vi "Get Listbox Text.vi"(8 "error in (no error)":errorcluster, 10 "bitfile path":path, 11 "Node Ptr":T1 format="%.0x") -> (0 "error out":errorcluster, 2 "Control Info":string[][](array[string]), 3 "Node Ptr out":T1 format="%.0x")   [LabVIEW 2013, in "PWM System Explorer.lvlib"]
uses:
  PWM System Explorer.lvlib
  <vilib>/NI Veristand/Custom Device API/Custom Device Item Ref.ctl
  Shared/Constants.vi
  <vilib>/regexp/Match Regular Expression.xnode
  Shared/PWM Shared.lvlib
  <vilib>/NI Veristand/Custom Device API/Custom Device API.lvlib
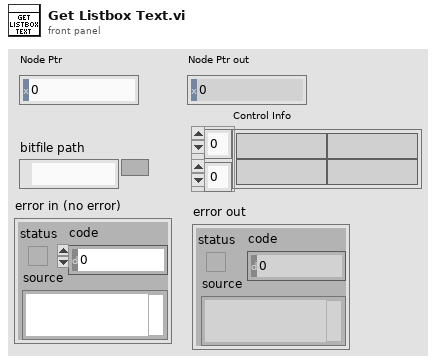
[diagram p1: front panel]
types:
  T1 = typedef "Custom Device API.lvlib/Custom Device Item Ref.ctl" = u64
  T2 = typedef "nirviReadCallControlInfo.ctl" = cluster{"names":string[], "indicator":bool[], "type descriptor":variant[], "size/rep":u32[], "top level type descriptor":variant[], "level":i32[], "class":string[], "address":i32[], "item orders":cluster{"order":u32[]}[], "name hierarchies":cluster{"name":string[]}[], "access may timeout":bool[], "from register node":bool[]}
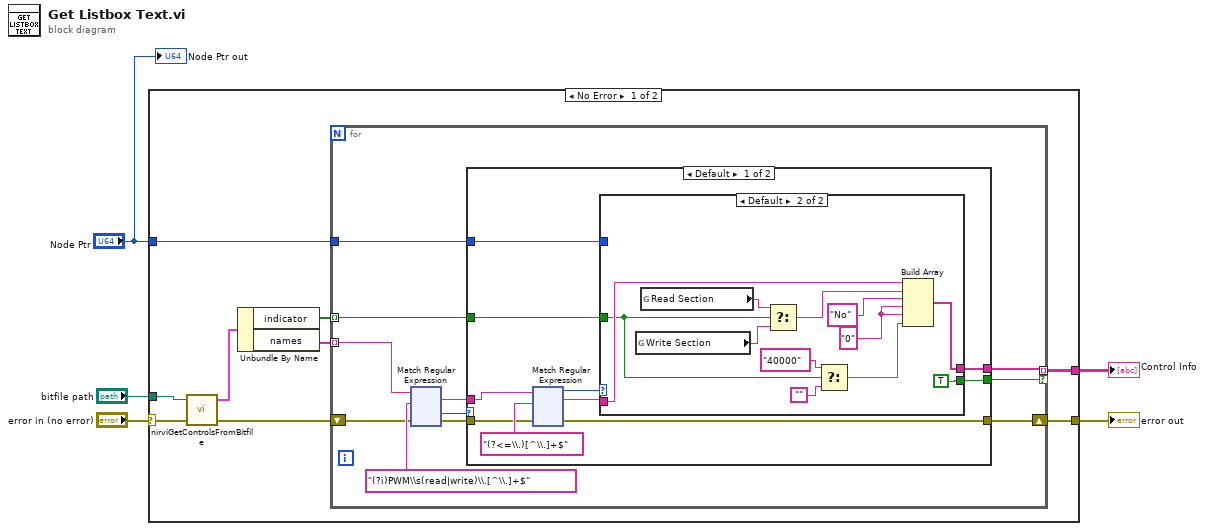
[diagram p0: block diagram]
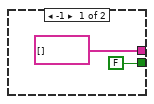
[diagram p2: hidden frame]
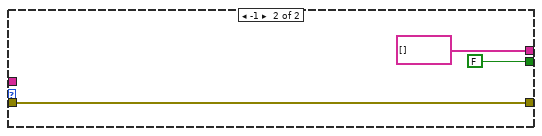
[diagram p3: hidden frame]
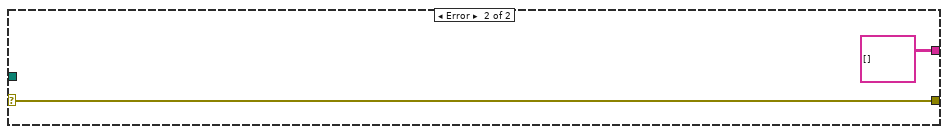
[diagram p4: hidden frame]
diagram:
  n1 = case shown="No Error" "error in (no error)" {
    selector: "error in (no error)" -> [w10 w282]
    tunnel: [w14 string[][] []] -> w5
    tunnel: "bitfile path" -> [w8 _]
    tunnel: [w11 w282] -> w2
    tunnel: "Node Ptr" -> [w6 _]
    frame No Error {
      n2 = call <vilib>:"nirviGetControlsFromBitfile.vi"("error in (no error)"=w10, "bitfile path"=w8) -> ("error out"=w9:errorcluster, "controls"=w12:T2)  [unwired: 2 in]
      n3 = Unbundle By Name(w12) -> ("indicator"=w13:bool[], "names"=w7:string[])
      n4 = for {
        tunnel: w7 -> [w25] mode=indexing
        tunnel: w13 -> [w21] mode=indexing
        tunnel: [w24] -> w14 mode=indexing if=w23
        shift-right: [w22] -> w11
        shift-left: w9 -> [w15]
        tunnel: w6 -> [w20]
        n5 = xnode "Match Regular Expression"("input string"=w25, "regular expression"="(?i)PWM\\s(read|write)\\.[^\\.]+$", "error in"=w15) -> ("whole match"=w17:string, "offset past match"=w19:i32, "error out"=w16:errorcluster)  [unwired: 3 in, 2 out]
        n6 = case shown="Default" w19 {
          tunnel: w21 -> [w35 _]
          tunnel: w17 -> [w30 _]
          tunnel: [w34 string[] []] -> w24
          tunnel: [w33 FALSE] -> w23
          tunnel: w20 -> [w28 _]
          tunnel: w16 -> [w27 w165]
          tunnel: [w26 w165] -> w22
          frame Default {
            n7 = xnode "Match Regular Expression"("input string"=w30, "regular expression"="(?<=\\.)[^\\.]+$", "error in"=w27) -> ("whole match"=w29:string, "offset past match"=w31:i32, "error out"=w26:errorcluster)  [unwired: 3 in, 2 out]
            n8 = case shown="Default" w31 {
              tunnel: w35 -> [_ w153]
              tunnel: w29 -> [_ w159]
              tunnel: [string[] [] w156] -> w34
              tunnel: [FALSE TRUE] -> w33
              tunnel: w28 -> [_ _]
              frame -1 {
              }
              frame Default {
                w157 = "0" ("regular expression")
                n9 = global read "Constants.vi" "Write Section"() -> (w162:string)
                n10 = global read "Constants.vi" "Read Section"() -> (w161:string)
                n11 = Select(t=w161, s=w153, f=w162) -> (s? t:f=w160:string)
                n12 = Select(t="40000" ("regular expression"), s=w153, f="" ("regular expression")) -> (s? t:f=w152:string)
                n13 = Build Array(w159, w160, "No" ("string"), w157, w157, w152) -> (w156:string[])
              }
            }
          }
          frame -1 {
          }
        }
      }
    }
    frame Error {
    }
  }
  "Control Info" <- w5
  "error out" <- w2
  "Node Ptr out" <- "Node Ptr"
